vi "ikine.vi"(8 "w":dbl min=-12.5664 max=12.5664 step=0.01, 11 "v":dbl min=-12.5664 max=12.5664 step=0.01) -> (0 "phi_r":dbl, 3 "phi_d":dbl)   [LabVIEW 2019]
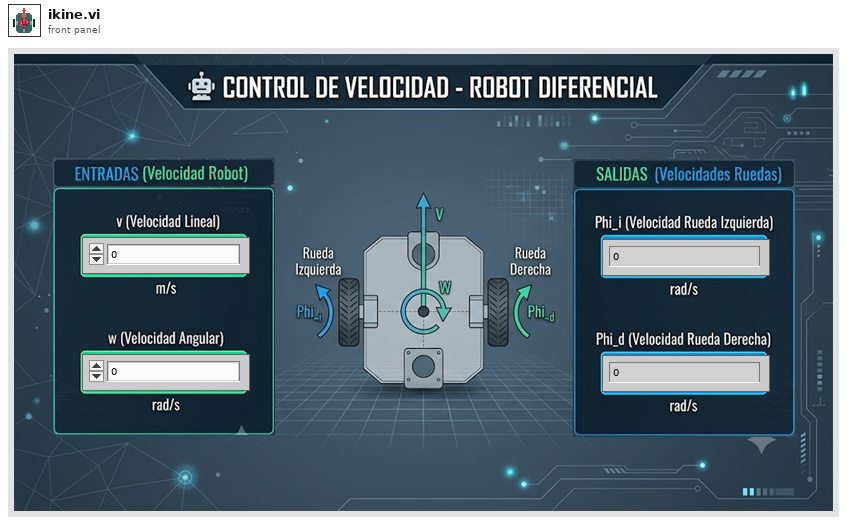
[diagram p1: front panel]
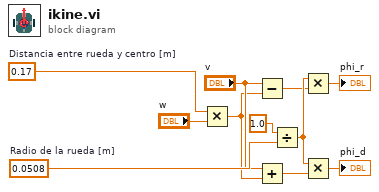
[diagram p0: block diagram]
diagram:
  w8 = 0.17  # Distancia entre rueda y centro [m]
  w9 = 0.0508  # Radio de la rueda [m]
  n1 = Multiply(x=w8, y="w") -> (x*y=w4:dbl)
  n2 = Subtract(x="v", y=w4) -> (x-y=w2:dbl)
  n3 = Add(x="v", y=w4) -> (x+y=w6:dbl)
  n4 = Divide(x=1.0 ("y"), y=w9) -> (x/y=w3:dbl)
  n5 = Multiply(x=w3, y=w2) -> (x*y=→"phi_r":dbl)
  n6 = Multiply(x=w3, y=w6) -> (x*y=→"phi_d":dbl)
